vi "b-fields many sensors tx ty.vi"(0 "magnet location tx ty BrV":T1, 7 "Magnetometer reading set":T2) -> (4 "mf - flat":dbl[](array[numeric]), 6 "pf - flat":dbl[](array[numeric]), 8 "derivative":dbl[][](array[numeric]), 13 "sensor0 prediction":dbl[](array[numeric]), 14 "sensor0 measured":dbl[](array[numeric]))   [LabVIEW 2017]
uses:
  typedefs/magnetomter reading set.ctl
  typedefs/magnet location tx ty.ctl
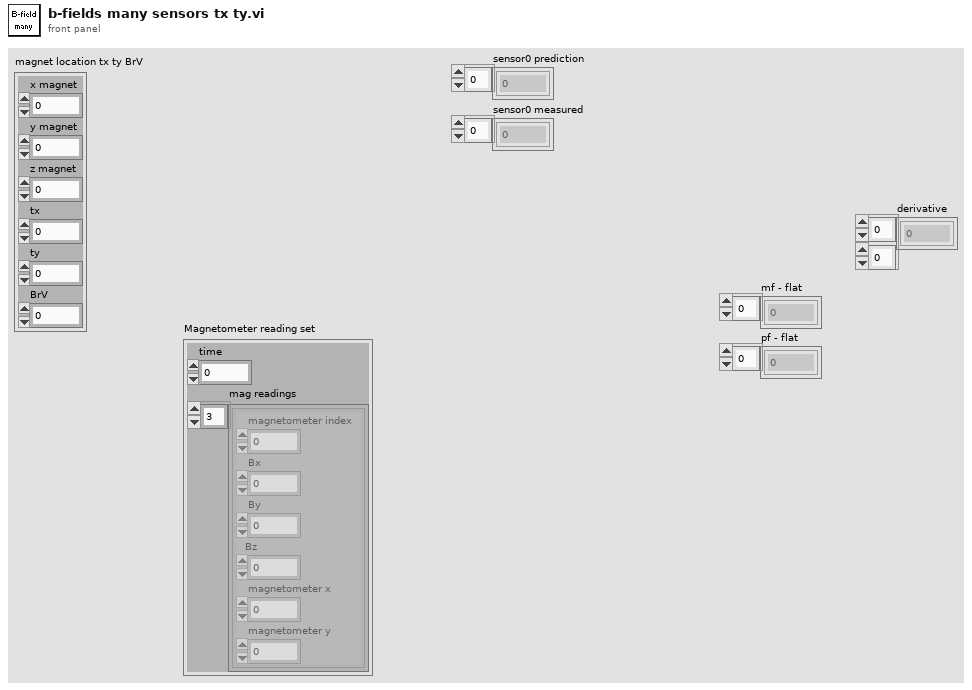
[diagram p1: front panel]
types:
  T1 = typedef "magnet location tx ty.ctl" = cluster{"x magnet":dbl, "y magnet":dbl, "z magnet":dbl, "tx":dbl, "ty":dbl, "BrV":dbl}
  T2 = typedef "magnetomter reading set.ctl" = cluster{"time":fxp<+,48,48>, "mag readings":cluster{"magnetometer index":dbl, "Bx":dbl, "By":dbl, "Bz":dbl, "magnetometer x":dbl, "magnetometer y":dbl}[]}
  T3 = cluster{"magnetometer index":dbl, "Bx":dbl, "By":dbl, "Bz":dbl, "magnetometer x":dbl, "magnetometer y":dbl}[]
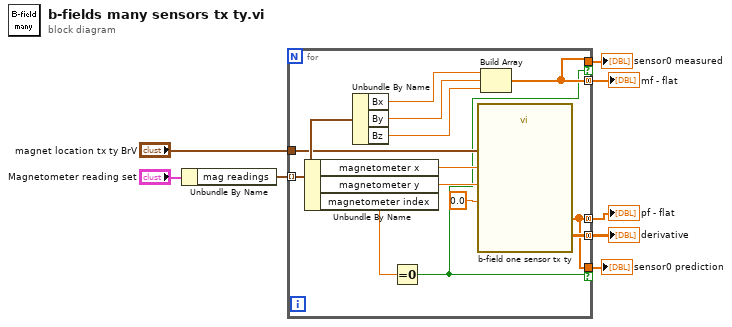
[diagram p0: block diagram]
diagram:
  n1 = Unbundle By Name("Magnetometer reading set") -> ("mag readings"=w8:T3)
  n2 = for {
    tunnel: w8 -> [w21] mode=indexing
    tunnel: [w10] -> w6 mode=concatenating
    tunnel: [w11] -> w5 mode=concatenating
    tunnel: "magnet location tx ty BrV" -> [w14]
    tunnel: [w13] -> w4 mode=concatenating
    tunnel: [w11] -> w2 if=w9
    tunnel: [w10] -> w1 if=w9
    n3 = Unbundle By Name(w21) -> ("magnetometer x"=w17:dbl, "magnetometer y"=w16:dbl, "magnetometer index"=w12:dbl)
    n4 = Unbundle By Name(w21) -> ("Bx"=w20:dbl, "By"=w19:dbl, "Bz"=w18:dbl)
    n5 = Equal To 0?(x=w12) -> (x = 0?=w9:bool)
    n6 = call "b-field one sensor tx ty.vi"("magnet location params"=w14, "x sensor"=w17, "y sensor"=w16, "z sensor"=0.0) -> ("Bx,By,Bz (uT)"=w11:dbl[], "dB (x,y,z, tx, ty, BrV)"=w13:dbl[][])  [unwired: 10 in]
    n7 = Build Array(w20, w19, w18) -> (w10:dbl[])
  }
  "mf - flat" <- w6
  "pf - flat" <- w5
  "derivative" <- w4
  "sensor0 prediction" <- w2
  "sensor0 measured" <- w1
